vi "ADD_RECORD.vi"(8 "error in (no error)":errorcluster caption="错误输入（无错误）", 11 "mes参数":string[](array[string])) -> (0 "error out":errorcluster caption="错误输出", 1 "body":string, 2 "出站成功":bool)   [LabVIEW 2015]
uses:
  Global.vi
panel:
  out "preasure":string="0"
  out "leak":string="0"
  out "failure_message":string="0"
  out "result":string="sn="
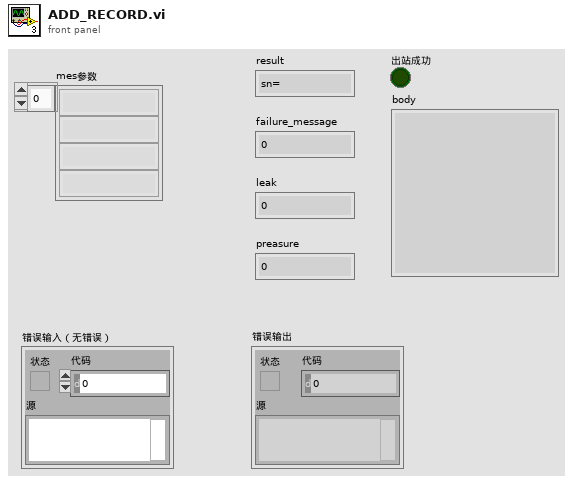
[diagram p1: front panel]
types:
  T1 = cluster{"URL":string, "audit_mode":string, "tsid":string, "model":string, "product":string, "test_station":string, "station_id":string, "test_station_name":string, "Webservice":string}
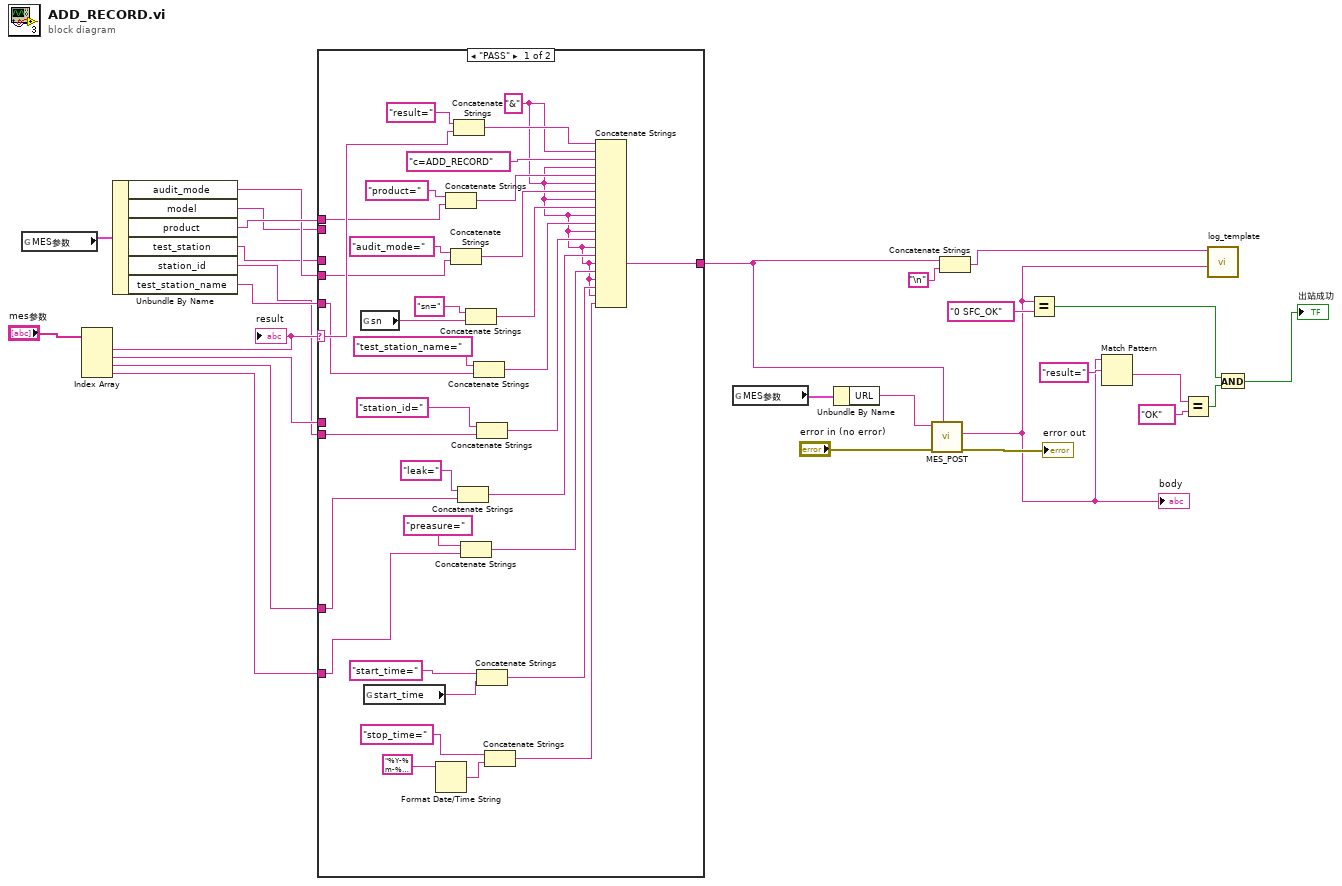
[diagram p0: block diagram]
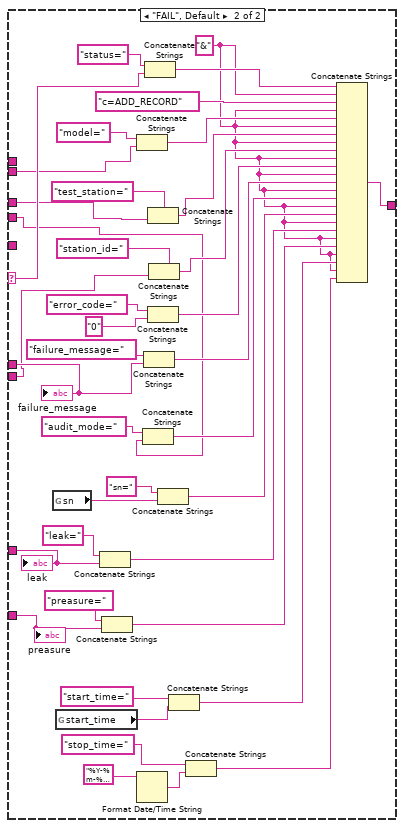
[diagram p2: hidden frame]
diagram:
  n1 = global read "Global.vi" "MES参数"() -> (w14:T1)
  n2 = Index Array(array="mes参数") -> (element #1=w18:string, element #2=w17:string, element #3=w16:string, element #4=w15:string)  [unwired: 4 in]
  "result" <- w18
  n3 = Unbundle By Name(w14) -> ("audit_mode"=w12:string, "model"=w9:string, "product"=w13:string, "test_station"=w8:string, "station_id"=w10:string, "test_station_name"=w11:string)
  n4 = case shown="\"PASS\"" w18 {
    selector: w18 -> [w59 w99]
    tunnel: [w60 w100] -> w23
    tunnel: w17 -> [_ w68]
    tunnel: w16 -> [w33 w67]
    tunnel: w15 -> [w31 w66]
    tunnel: w13 -> [w38 _]
    tunnel: w12 -> [w37 w62]
    tunnel: w11 -> [w36 _]
    tunnel: w10 -> [w35 w63]
    tunnel: w9 -> [_ w65]
    tunnel: w8 -> [_ w64]
    frame "PASS" {
      w28 = "&"
      n5 = global read "Global.vi" "sn"() -> (w51:string)
      n6 = global read "Global.vi" "start_time"() -> (w41:string)
      n7 = Format Date/Time String(time format string (%c)="%Y-%m-%d %H:%M:%S" ("EndTime")) -> (date/time string=w43:string)  [unwired: 2 in]
      n8 = Concatenate Strings("product=", w38) -> (w54:string)
      n9 = Concatenate Strings("audit_mode=", w37) -> (w52:string)
      n10 = Concatenate Strings("result=", w59) -> (w56:string)
      n11 = Concatenate Strings("leak=", w33) -> (w30:string)
      n12 = Concatenate Strings("preasure=", w31) -> (w29:string)
      n13 = Concatenate Strings("sn=", w51) -> (w49:string)
      n14 = Concatenate Strings("test_station_name=", w36) -> (w48:string)
      n15 = Concatenate Strings("station_id=", w35) -> (w46:string)
      n16 = Concatenate Strings("start_time=", w41) -> (w40:string)
      n17 = Concatenate Strings("stop_time=", w43) -> (w39:string)
      n18 = Concatenate Strings(w56, w28, "c=ADD_RECORD", w28, w54, w28, w52, w28, w49, w28, w48, w28, w46, w28, w30, w28, w29, w28, w40, w28, w39) -> (w60:string)
    }
    frame "FAIL", Default {
      w70 = "&"
      n19 = global read "Global.vi" "sn"() -> (w79:string)
      n20 = global read "Global.vi" "start_time"() -> (w88:string)
      n21 = Concatenate Strings("leak=", w67) -> (w73:string)
      n22 = Concatenate Strings("preasure=", w66) -> (w72:string)
      n23 = Concatenate Strings("model=", w65) -> (w94:string)
      n24 = Format Date/Time String(time format string (%c)="%Y-%m-%d %H:%M:%S" ("EndTime")) -> (date/time string=w90:string)  [unwired: 2 in]
      n25 = Concatenate Strings("audit_mode=", w62) -> (w77:string)
      n26 = Concatenate Strings("failure_message=", w68) -> (w81:string)
      n27 = Concatenate Strings("status=", w99) -> (w96:string)
      n28 = Concatenate Strings("test_station=", w64) -> (w87:string)
      n29 = Concatenate Strings("error_code=", "0") -> (w83:string)
      n30 = Concatenate Strings("station_id=", w63) -> (w86:string)
      n31 = Concatenate Strings("sn=", w79) -> (w76:string)
      n32 = Concatenate Strings("start_time=", w88) -> (w71:string)
      n33 = Concatenate Strings("stop_time=", w90) -> (w69:string)
      n34 = Concatenate Strings(w96, w70, "c=ADD_RECORD", w70, w94, w70, w87, w70, w86, w70, w83, w70, w81, w70, w77, w70, w76, w70, w73, w70, w72, w70, w71, w70, w69) -> (w100:string)
      "failure_message" <- w68
      "leak" <- w67
      "preasure" <- w66
    }
  }
  n35 = global read "Global.vi" "MES参数"() -> (w25:T1)
  n36 = Unbundle By Name(w25) -> ("URL"=w21:string)
  n37 = call "MES_POST.vi"("DATA"=w23, "错误输入（无错误）"="error in (no error)", "URL"=w21) -> ("错误输出"=→"error out":errorcluster, "body"=w6:string)  [unwired: 6 in, 1 out]
  "body" <- w6
  n38 = Concatenate Strings(w23, "\n") -> (w20:string)
  n39 = Equal?(x=w6, y="0 SFC_OK") -> (x = y?=w2:bool)
  n40 = Match Pattern(string=w6, regular expression="result=" ("正则表达式")) -> (after substring=w4:string)  [unwired: 1 in, 3 out]
  n41 = Equal?(x=w4, y="OK") -> (x = y?=w3:bool)
  n42 = call "log_template.vi"("接收报文"=w6, "发送报文"=w20) -> ()  [unwired: 10 in]
  n43 = And(x=w2, y=w3) -> (x .and. y?=→"出站成功":bool)
